vi "SEND_Probe.vi"(1 "Messenging.lvlib:Send.lvclass":refnum<class "Send.lvclass">) -> (0 "Boolean":bool)   [LabVIEW 2011, in "Messenging.lvlib"]
uses:
  Messenging.lvlib
  Interprocess Messenger/Send/Send.lvclass
panel:
  out "Description":string
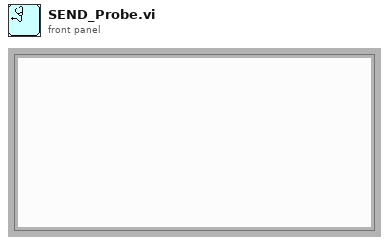
[diagram p1: front panel]
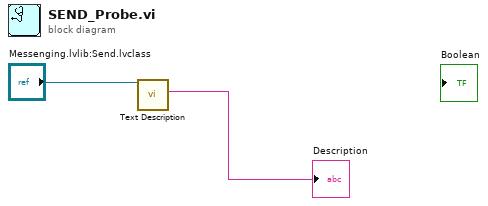
[diagram p0: block diagram]
diagram:
  n1 = call-dynamic "Text Description.vi"("Send in"="Messenging.lvlib:Send.lvclass") -> ("Description"=→"Description":string)  [unwired: 10 out]
